vi "Stepper master control.vi"(8 "Speed":dbl, 9 "Pos":cluster{dbl, dbl, dbl, dbl, dbl, dbl, dbl, dbl}, 11 "FPGA VI Reference In":refnum<k20>) -> (2 "0?":bool)   [LabVIEW 2019]
uses:
  <vilib>/Utility/error.llb/Error Cluster From Error Code.vi
  <vilib>/rvi/errors/niLvFpgaAdjustHostInterfaceError.vi
  <vilib>/rvi/interface/nirviReadWriteControl/nirviReadWriteControl.xnode
  NiFpgaLv.dll
  <vilib>/rvi/interface/Simulation/niFpgaSimulationCallBeginRW.vi
panel:
  # "1"
  # "2"
  # "3"
  # "4"
  # "5"
  # "6"
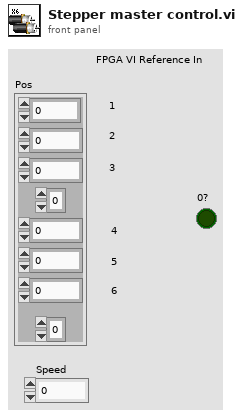
[diagram p1: front panel]
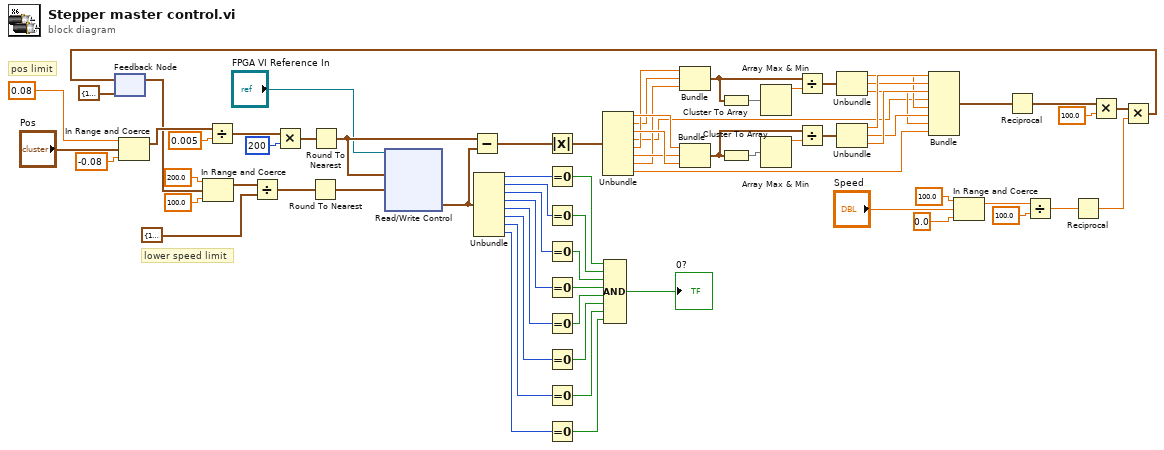
[diagram p0: block diagram]
diagram:
  # "lower speed limit"
  # "pos limit"
  n1 = feedback #1(cluster{dbl, dbl, dbl, dbl, dbl, dbl, dbl, dbl} {100.0, 100.0, 100.0, 100.0, 100.0, 100.0, 100.0, 100.0}) -> (w36:cluster{dbl, dbl, dbl, dbl, dbl, dbl, dbl, dbl})
  n2 = In Range and Coerce(upper limit=0.08, x="Pos", lower limit=-0.08) -> (coerced(x)=w62:cluster{dbl, dbl, dbl, dbl, dbl, dbl, dbl, dbl})  [unwired: 1 out]
  n3 = In Range and Coerce(upper limit=200.0, x=w36, lower limit=100.0) -> (coerced(x)=w7:cluster{dbl, dbl, dbl, dbl, dbl, dbl, dbl, dbl})  [unwired: 1 out]
  n4 = Divide(x=w62, y=0.005) -> (x/y=w67:cluster{dbl, dbl, dbl, dbl, dbl, dbl, dbl, dbl})
  n5 = Divide(x=w7, y=cluster{dbl, dbl, dbl, dbl, dbl, dbl, dbl, dbl} {1.0, 10.0, 1.0, 1.0, 1.0, 1.0, 1.0, 1.0}) -> (x/y=w6:cluster{dbl, dbl, dbl, dbl, dbl, dbl, dbl, dbl})
  n6 = Multiply(x=w67, y=i16 200) -> (x*y=w71:cluster{dbl, dbl, dbl, dbl, dbl, dbl, dbl, dbl})
  n7 = Round To Nearest(number=w6) -> (nearest integer value=w4:cluster{dbl, dbl, dbl, dbl, dbl, dbl, dbl, dbl})
  n8 = Round To Nearest(number=w71) -> (nearest integer value=w3:cluster{dbl, dbl, dbl, dbl, dbl, dbl, dbl, dbl})
  n9 = xnode "Read/Write Control"("FPGA VI Reference In"="FPGA VI Reference In", "Steps"=w3, "Skipper"=w4) -> ("Cluster"=w1:cluster{i16, i16, i16, i16, i16, i16, i16, i16})  [unwired: 1 in, 2 out]
  n10 = Subtract(x=w3, y=w1) -> (x-y=w65:cluster{dbl, dbl, dbl, dbl, dbl, dbl, dbl, dbl})
  n11 = Unbundle(w1) -> (w53:i16, w52:i16, w51:i16, w50:i16, w49:i16, w48:i16, w47:i16, w46:i16)
  n12 = Absolute Value(x=w65) -> (abs(x)=w32:cluster{dbl, dbl, dbl, dbl, dbl, dbl, dbl, dbl})
  n13 = Equal To 0?(x=w53) -> (x = 0?=w45:bool)
  n14 = Equal To 0?(x=w52) -> (x = 0?=w44:bool)
  n15 = Equal To 0?(x=w51) -> (x = 0?=w43:bool)
  n16 = Equal To 0?(x=w50) -> (x = 0?=w42:bool)
  n17 = Equal To 0?(x=w49) -> (x = 0?=w41:bool)
  n18 = Equal To 0?(x=w48) -> (x = 0?=w40:bool)
  n19 = Equal To 0?(x=w47) -> (x = 0?=w39:bool)
  n20 = Equal To 0?(x=w46) -> (x = 0?=w38:bool)
  n21 = Unbundle(w32) -> (w24:dbl, w16:dbl, w23:dbl, w12:dbl, w18:dbl, w22:dbl, w17:dbl, w25:dbl)
  n22 = Compound Arithmetic op=AND(w45, w44, w43, w42, w41, w40, w39, w38) -> (→"0?":bool)
  n23 = Bundle(w18, w16, w17) -> (w10:cluster{dbl, dbl, dbl})  [unwired: 1 in]
  n24 = Bundle(w24, w22, w23) -> (w11:cluster{dbl, dbl, dbl})  [unwired: 1 in]
  n25 = Cluster To Array(cluster=w10) -> (array=w30:dbl[])
  n26 = Cluster To Array(cluster=w11) -> (array=w31:dbl[])
  n27 = Array Max & Min(array=w30) -> (max value=w29:dbl)  [unwired: 3 out]
  n28 = Array Max & Min(array=w31) -> (max value=w28:dbl)  [unwired: 3 out]
  n29 = Divide(x=w10, y=w29) -> (x/y=w26:cluster{dbl, dbl, dbl})
  n30 = Divide(x=w11, y=w28) -> (x/y=w27:cluster{dbl, dbl, dbl})
  n31 = Unbundle(w26) -> (w14:dbl, w15:dbl, w13:dbl)
  n32 = Unbundle(w27) -> (w21:dbl, w19:dbl, w20:dbl)
  n33 = Bundle(w21, w15, w20, w12, w14, w19, w13, w25) -> (w9:cluster{dbl, dbl, dbl, dbl, dbl, dbl, dbl, dbl})  [unwired: 1 in]
  n34 = In Range and Coerce(upper limit=100.0, x="Speed", lower limit=0.0) -> (coerced(x)=w35:dbl)  [unwired: 1 out]
  n35 = Reciprocal(x=w9) -> (1/x=w64:cluster{dbl, dbl, dbl, dbl, dbl, dbl, dbl, dbl})
  n36 = Divide(x=w35, y=100.0) -> (x/y=w57:dbl)
  n37 = Reciprocal(x=w57) -> (1/x=w54:dbl)
  n38 = Multiply(x=w64, y=100.0) -> (x*y=w56:cluster{dbl, dbl, dbl, dbl, dbl, dbl, dbl, dbl})
  n39 = Multiply(x=w56, y=w54) -> (x*y=w55:cluster{dbl, dbl, dbl, dbl, dbl, dbl, dbl, dbl})
  n40 = feedback-in #1(w55) -> ()
